vi "Lab Panel V5.31.vi"() -> ()   [LabVIEW 2017] (continued)
                            n1780 = local write "RUN LAB05-2"(w3330) -> ()
                            n1781 = local write "O/I  LAB05-2"(w3330) -> ()
                            n1782 = local write "run lab05-2"(w3330) -> ()
                            n1783 = local write "DISP LAB05-2"(w3333) -> ()
                          }
                          frame #1 {
                            n1784 = TDMS Close(11:w3334) -> (0:w3335:errorcluster)  [unwired: 1 in, 1 out]
                            n1785 = local write "data file error"(w3335) -> ()
                          }
                          frame #2 {
                            n1786 = stacked-sequence {
                              tunnel: "LAB05-2" -> [w3343 w3349]
                              tunnel: w3340 -> [_ w3348]
                              tunnel: w3339 -> [_ w3347]
                              tunnel: w3338 -> [_ w3346]
                              tunnel: w3337 -> [_ w3345]
                              tunnel: w3336 -> [_ w3344]
                              frame #0 {
                                n1787 = call "sub vi - defrag tdms v1.vi"("panel id"=w3343) -> ("error out"=w3342:errorcluster)  [unwired: 10 in]
                                n1788 = local write "data file error"(w3342) -> ()
                              }
                              frame #1 {
                                n1789 = Bundle("STATUS"=w3348, "OUT SERVER ADDRESS"=w3347, "FROM ACCOUNT"=w3346, "Mail Test File To:"=w3345, "Mail Test Fail"=w3344) -> (w3351:T29)  [unwired: 1 in]
                                n1790 = call "Save data file (pass-fail) v5.vi"("Input Cluster"=w3351, "panel id"=w3349) -> ("network file save error"=w3350:errorcluster)  [unwired: 8 in, 1 out]
                                n1791 = local write "data file error"(w3350) -> ()
                              }
                            }
                          }
                        }
                      }
                    }
                  }
                }
              }
            }
            n1792 = global write "Global display 2.vi" "Mail test file to:"(w2858) -> ()
            n1793 = local read "Network Directory"() -> (w2864:path)
            n1794 = global write "Global 1.vi" "Network Drive"(w2864) -> ()
          }
          frame #8 {
            # "disable functions"
            n1795 = stacked-sequence {
              tunnel: w3361 -> [w3375 _ w3432]
              tunnel: w3360 -> [w3370 _ w3431]
              tunnel: w3359 -> [w3369 _ w3430]
              tunnel: w3358 -> [w3367 _ w3429]
              tunnel: w3357 -> [w3368 _ w3428]
              tunnel: w3356 -> [_ w3392 w3427]
              tunnel: w3355 -> [_ w3393 w3426]
              tunnel: w3354 -> [_ w3394 w3425]
              tunnel: w3353 -> [_ w3395 w3424]
              tunnel: w3352 -> [_ w3396 w3423]
              frame #0 {
                n1796 = Select(t=2, s=w3367, f=0) -> (s? t:f=w3363:i32)
                n1797 = Select(t=2, s=w3369, f=0) -> (s? t:f=w3364:i32)
                n1798 = Select(t=2, s=w3368, f=0) -> (s? t:f=w3362:i32)
                n1799 = Select(t=2, s=w3375, f=0) -> (s? t:f=w3366:i32)
                n1800 = Select(t=2, s=w3370, f=0) -> (s? t:f=w3365:i32)
                n1801 = property on="SELECT LAB02-2" class="RadioBtnsControl (strict)"("DisabledEnum"=w3363) -> ()  [unwired: 2 in, 2 out]
                n1802 = property on="SELECT LAB02-1" class="RadioBtnsControl (strict)"("DisabledEnum"=w3364) -> ()  [unwired: 2 in, 2 out]
                n1803 = property on="SELECT LAB03-1" class="RadioBtnsControl (strict)"("DisabledEnum"=w3362) -> ()  [unwired: 2 in, 2 out]
                n1804 = property on="SELECT LAB01-1" class="RadioBtnsControl (strict)"("DisabledEnum"=w3366) -> ()  [unwired: 2 in, 2 out]
                n1805 = property on="SELECT LAB01-2" class="RadioBtnsControl (strict)"("DisabledEnum"=w3365) -> ()  [unwired: 2 in, 2 out]
                n1806 = Not(x=w3375) -> (.not. x?=w3376:bool)
                n1807 = property on="RESULT LAB01-1" class="Bool (strict)"("Visible"=w3376) -> ()  [unwired: 2 in, 2 out]
                n1808 = Not(x=w3370) -> (.not. x?=w3374:bool)
                n1809 = Not(x=w3369) -> (.not. x?=w3373:bool)
                n1810 = Not(x=w3367) -> (.not. x?=w3372:bool)
                n1811 = property on="RESULT LAB01-2" class="Bool (strict)"("Visible"=w3374) -> ()  [unwired: 2 in, 2 out]
                n1812 = Not(x=w3368) -> (.not. x?=w3371:bool)
                n1813 = property on="RESULT LAB02-1" class="Bool (strict)"("Visible"=w3373) -> ()  [unwired: 2 in, 2 out]
                n1814 = property on="RESULT LAB02-2" class="Bool (strict)"("Visible"=w3372) -> ()  [unwired: 2 in, 2 out]
                n1815 = property on="RESULT LAB03-1" class="Bool (strict)"("Visible"=w3371) -> ()  [unwired: 2 in, 2 out]
                n1816 = property on="SET LAB01-1" class="Clust (strict)"("DisabledEnum"=w3366) -> ()  [unwired: 2 in, 2 out]
                n1817 = property on="SET LAB01-2" class="Clust (strict)"("DisabledEnum"=w3365) -> ()  [unwired: 2 in, 2 out]
                n1818 = property on="SET LAB02-1" class="Clust (strict)"("DisabledEnum"=w3364) -> ()  [unwired: 2 in, 2 out]
                n1819 = property on="SET LAB02-2" class="Clust (strict)"("DisabledEnum"=w3363) -> ()  [unwired: 2 in, 2 out]
                n1820 = property on="SET LAB03-1" class="Clust (strict)"("DisabledEnum"=w3362) -> ()  [unwired: 2 in, 2 out]
                n1821 = property on="O/I  LAB01-1" class="Bool (strict)"("DisabledEnum"=w3366) -> ()  [unwired: 2 in, 2 out]
                n1822 = property on="O/I  LAB01-2" class="Bool (strict)"("DisabledEnum"=w3365) -> ()  [unwired: 2 in, 2 out]
                n1823 = property on="O/I  LAB02-1" class="Bool (strict)"("DisabledEnum"=w3364) -> ()  [unwired: 2 in, 2 out]
                n1824 = property on="O/I  LAB02-2" class="Bool (strict)"("DisabledEnum"=w3363) -> ()  [unwired: 2 in, 2 out]
                n1825 = property on="O/I  LAB03-1" class="Bool (strict)"("DisabledEnum"=w3362) -> ()  [unwired: 2 in, 2 out]
              }
              frame #1 {
                n1826 = Select(t=2, s=w3396, f=0) -> (s? t:f=w3387:i32)
                n1827 = Select(t=2, s=w3395, f=0) -> (s? t:f=w3388:i32)
                n1828 = Select(t=2, s=w3392, f=0) -> (s? t:f=w3391:i32)
                n1829 = Select(t=2, s=w3393, f=0) -> (s? t:f=w3390:i32)
                n1830 = Select(t=2, s=w3394, f=0) -> (s? t:f=w3389:i32)
                n1831 = property on="SELECT LAB05-2" class="RadioBtnsControl (strict)"("DisabledEnum"=w3387) -> ()  [unwired: 2 in, 2 out]
                n1832 = property on="SELECT LAB05-1" class="RadioBtnsControl (strict)"("DisabledEnum"=w3388) -> ()  [unwired: 2 in, 2 out]
                n1833 = property on="SELECT LAB03-2" class="RadioBtnsControl (strict)"("DisabledEnum"=w3391) -> ()  [unwired: 2 in, 2 out]
                n1834 = property on="SELECT LAB04-1" class="RadioBtnsControl (strict)"("DisabledEnum"=w3390) -> ()  [unwired: 2 in, 2 out]
                n1835 = property on="SELECT LAB04-2" class="RadioBtnsControl (strict)"("DisabledEnum"=w3389) -> ()  [unwired: 2 in, 2 out]
                n1836 = property on="SET LAB05-2" class="Clust (strict)"("DisabledEnum"=w3387) -> ()  [unwired: 2 in, 2 out]
                n1837 = property on="SET LAB05-1" class="Clust (strict)"("DisabledEnum"=w3388) -> ()  [unwired: 2 in, 2 out]
                n1838 = property on="SET LAB03-2" class="Clust (strict)"("DisabledEnum"=w3391) -> ()  [unwired: 2 in, 2 out]
                n1839 = property on="SET LAB04-1" class="Clust (strict)"("DisabledEnum"=w3390) -> ()  [unwired: 2 in, 2 out]
                n1840 = property on="SET LAB04-2" class="Clust (strict)"("DisabledEnum"=w3389) -> ()  [unwired: 2 in, 2 out]
                n1841 = property on="O/I  LAB05-2" class="Bool (strict)"("DisabledEnum"=w3387) -> ()  [unwired: 2 in, 2 out]
                n1842 = property on="O/I  LAB05-1" class="Bool (strict)"("DisabledEnum"=w3388) -> ()  [unwired: 2 in, 2 out]
                n1843 = property on="O/I  LAB04-1" class="Bool (strict)"("DisabledEnum"=w3390) -> ()  [unwired: 2 in, 2 out]
                n1844 = property on="O/I  LAB04-2" class="Bool (strict)"("DisabledEnum"=w3389) -> ()  [unwired: 2 in, 2 out]
                n1845 = property on="O/I  LAB03-2" class="Bool (strict)"("DisabledEnum"=w3391) -> ()  [unwired: 2 in, 2 out]
                n1846 = Not(x=w3396) -> (.not. x?=w3397:bool)
                n1847 = Not(x=w3395) -> (.not. x?=w3398:bool)
                n1848 = Not(x=w3394) -> (.not. x?=w3399:bool)
                n1849 = property on="RESULT LAB05-2" class="Bool (strict)"("Visible"=w3397) -> ()  [unwired: 2 in, 2 out]
                n1850 = property on="RESULT LAB05-1" class="Bool (strict)"("Visible"=w3398) -> ()  [unwired: 2 in, 2 out]
                n1851 = Not(x=w3393) -> (.not. x?=w3400:bool)
                n1852 = property on="RESULT LAB04-2" class="Bool (strict)"("Visible"=w3399) -> ()  [unwired: 2 in, 2 out]
                n1853 = Not(x=w3392) -> (.not. x?=w3401:bool)
                n1854 = property on="RESULT LAB04-1" class="Bool (strict)"("Visible"=w3400) -> ()  [unwired: 2 in, 2 out]
                n1855 = property on="RESULT LAB03-2" class="Bool (strict)"("Visible"=w3401) -> ()  [unwired: 2 in, 2 out]
              }
              frame #2 {
                # "disable calibrate if any test running"
                n1856 = Or(x=w3424, y=w3423) -> (x .or. y?=w3417:bool)
                n1857 = Or(x=w3426, y=w3425) -> (x .or. y?=w3419:bool)
                n1858 = Or(x=w3430, y=w3429) -> (x .or. y?=w3421:bool)
                n1859 = Or(x=w3428, y=w3427) -> (x .or. y?=w3420:bool)
                n1860 = Or(x=w3432, y=w3431) -> (x .or. y?=w3422:bool)
                n1861 = Or(x=w3420, y=w3419) -> (x .or. y?=w3418:bool)
                n1862 = Or(x=w3422, y=w3421) -> (x .or. y?=w3416:bool)
                n1863 = Or(x=w3418, y=w3417) -> (x .or. y?=w3415:bool)
                n1864 = Or(x=w3416, y=w3415) -> (x .or. y?=w3412:bool)
                "Any Test Running" <- w3412
                n1865 = case shown="False" w3412 {
                  tunnel: [0 2] -> w3414
                  frame False {
                  }
                  frame True {
                  }
                }
                n1866 = property on="JIG TEST" class="Clust (strict)"("DisabledEnum"=w3414) -> ()  [unwired: 2 in, 2 out]
                n1867 = property on="Network Directory" class="Path"("DisabledEnum"=w3414) -> ()  [unwired: 2 in, 2 out]
                n1868 = property on="MAIL SETTINGS" class="Clust (strict)"("DisabledEnum"=w3414) -> ()  [unwired: 2 in, 2 out]
                n1869 = property on="SET (cal)" class="Bool (strict)"("DisabledEnum"=w3414) -> ()  [unwired: 2 in, 2 out]
                n1870 = property on="ADMIN" class="Bool (strict)"("DisabledEnum"=0) -> ()  [unwired: 2 in, 2 out]
              }
            }
          }
          frame #9 {
            # "Note : JIG LAB0X-N   are written to digital I/O in frame 11"
            # "Drive jigs"
            n1871 = stacked-sequence {
              frame #0 {
                # "jig on"
                n1872 = local read "jig cycle"() -> (w3440:dbl)
                n1873 = property on="JIG TEST" class="Clust (strict)"() -> ("DisabledEnum"=w3437:T17)  [unwired: 2 in, 2 out]
                n1874 = Equal?(x=w3437, y=2) -> (x = y?=w3436:bool)
                n1875 = Equal?(x=w3440, y=0) -> (x = y?=w3438:bool)
                n1876 = And(x=w3438, y=w3436) -> (x .and. y?=w3435:bool)
                n1877 = case shown="True" w3435 {
                  frame False {
                  }
                  frame True {
                    n1878 = local read "run lab01-2"() -> (w3450:bool)
                    n1879 = local read "run lab01-1"() -> (w3451:bool)
                    n1880 = local read "run lab02-1"() -> (w3449:bool)
                    n1881 = local read "run lab02-2"() -> (w3448:bool)
                    n1882 = local read "run lab03-1"() -> (w3447:bool)
                    n1883 = local read "run lab03-2"() -> (w3446:bool)
                    n1884 = local read "run lab04-1"() -> (w3445:bool)
                    n1885 = local read "run lab04-2"() -> (w3444:bool)
                    n1886 = local read "run lab05-1"() -> (w3443:bool)
                    n1887 = local read "run lab05-2"() -> (w3442:bool)
                    n1888 = local write "JIG LAB01-2"(w3450) -> ()
                    n1889 = local write "JIG LAB03-2"(w3446) -> ()
                    n1890 = local write "JIG LAB01-1"(w3451) -> ()
                    n1891 = local write "JIG LAB02-1"(w3449) -> ()
                    n1892 = local write "JIG LAB02-2"(w3448) -> ()
                    n1893 = local write "JIG LAB03-1"(w3447) -> ()
                    n1894 = local write "JIG LAB04-1"(w3445) -> ()
                    n1895 = local write "JIG LAB04-2"(w3444) -> ()
                    n1896 = local write "JIG LAB05-1"(w3443) -> ()
                    n1897 = local write "JIG LAB05-2"(w3442) -> ()
                  }
                }
              }
              frame #1 {
                # "jig off"
                n1898 = local read "jig cycle"() -> (w3458:dbl)
                n1899 = local read "on loops"() -> (w3457:dbl)
                n1900 = property on="JIG TEST" class="Clust (strict)"() -> ("DisabledEnum"=w3456:T17)  [unwired: 2 in, 2 out]
                n1901 = Equal?(x=w3456, y=2) -> (x = y?=w3454:bool)
                n1902 = Equal?(x=w3458, y=w3457) -> (x = y?=w3453:bool)
                n1903 = And(x=w3453, y=w3454) -> (x .and. y?=w3452:bool)
                n1904 = case shown="True" w3452 {
                  frame False {
                  }
                  frame True {
                    w3509 = FALSE
                    w3510 = TRUE
                    w3508 = 2
                    n1905 = local read "SELECT LAB05-2"() -> (w3499:T3)
                    n1906 = local read "SELECT LAB04-2"() -> (w3501:T3)
                    n1907 = local read "SELECT LAB04-1"() -> (w3502:T3)
                    n1908 = local read "SELECT LAB05-1"() -> (w3500:T3)
                    n1909 = local read "SELECT LAB03-2"() -> (w3503:T3)
                    n1910 = local read "SELECT LAB02-1"() -> (w3506:T3)
                    n1911 = local read "SELECT LAB03-1"() -> (w3504:T3)
                    n1912 = local read "SELECT LAB02-2"() -> (w3505:T3)
                    n1913 = local read "SELECT LAB01-2"() -> (w3507:T3)
                    n1914 = local read "run lab05-1"() -> (w3469:bool)
                    n1915 = local read "run lab05-2"() -> (w3468:bool)
                    n1916 = local read "run lab04-2"() -> (w3470:bool)
                    n1917 = local read "SELECT LAB01-1"() -> (w3511:T3)
                    n1918 = local read "run lab04-1"() -> (w3471:bool)
                    n1919 = local read "run lab01-1"() -> (w3487:bool)
                    n1920 = local read "run lab01-2"() -> (w3476:bool)
                    n1921 = local read "run lab03-2"() -> (w3472:bool)
                    n1922 = local read "run lab03-1"() -> (w3473:bool)
                    n1923 = local read "run lab02-1"() -> (w3475:bool)
                    n1924 = local read "run lab02-2"() -> (w3474:bool)
                    n1925 = Equal?(x=w3508, y=w3504) -> (x = y?=w3482:bool)
                    n1926 = Equal?(x=w3508, y=w3503) -> (x = y?=w3481:bool)
                    n1927 = Equal?(x=w3508, y=w3502) -> (x = y?=w3480:bool)
                    n1928 = Equal?(x=w3508, y=w3501) -> (x = y?=w3479:bool)
                    n1929 = Equal?(x=w3508, y=w3500) -> (x = y?=w3478:bool)
                    n1930 = Equal?(x=w3508, y=w3499) -> (x = y?=w3477:bool)
                    n1931 = Equal?(x=w3508, y=w3511) -> (x = y?=w3488:bool)
                    n1932 = Equal?(x=w3508, y=w3506) -> (x = y?=w3484:bool)
                    n1933 = Equal?(x=w3508, y=w3505) -> (x = y?=w3483:bool)
                    n1934 = Equal?(x=w3508, y=w3507) -> (x = y?=w3485:bool)
                    n1935 = And(x=w3479, y=w3470) -> (x .and. y?=w3461:bool)
                    n1936 = And(x=w3482, y=w3473) -> (x .and. y?=w3464:bool)
                    n1937 = And(x=w3480, y=w3471) -> (x .and. y?=w3462:bool)
                    n1938 = And(x=w3477, y=w3468) -> (x .and. y?=w3459:bool)
                    n1939 = And(x=w3483, y=w3474) -> (x .and. y?=w3465:bool)
                    n1940 = And(x=w3481, y=w3472) -> (x .and. y?=w3463:bool)
                    n1941 = And(x=w3478, y=w3469) -> (x .and. y?=w3460:bool)
                    n1942 = And(x=w3485, y=w3476) -> (x .and. y?=w3467:bool)
                    n1943 = And(x=w3488, y=w3487) -> (x .and. y?=w3486:bool)
                    n1944 = And(x=w3484, y=w3475) -> (x .and. y?=w3466:bool)
                    n1945 = Select(t=w3510, s=w3486, f=w3509) -> (s? t:f=w3489:bool)
                    n1946 = Select(t=w3510, s=w3467, f=w3509) -> (s? t:f=w3490:bool)
                    n1947 = Select(t=w3510, s=w3466, f=w3509) -> (s? t:f=w3491:bool)
                    n1948 = Select(t=w3510, s=w3465, f=w3509) -> (s? t:f=w3492:bool)
                    n1949 = Select(t=w3510, s=w3464, f=w3509) -> (s? t:f=w3493:bool)
                    n1950 = Select(t=w3510, s=w3463, f=w3509) -> (s? t:f=w3494:bool)
                    n1951 = Select(t=w3510, s=w3462, f=w3509) -> (s? t:f=w3495:bool)
                    n1952 = Select(t=w3510, s=w3461, f=w3509) -> (s? t:f=w3496:bool)
                    n1953 = Select(t=w3510, s=w3460, f=w3509) -> (s? t:f=w3497:bool)
                    n1954 = Select(t=w3510, s=w3459, f=w3509) -> (s? t:f=w3498:bool)
                    n1955 = local write "JIG LAB03-2"(w3494) -> ()
                    n1956 = local write "JIG LAB02-1"(w3491) -> ()
                    n1957 = local write "JIG LAB02-2"(w3492) -> ()
                    n1958 = local write "JIG LAB01-2"(w3490) -> ()
                    n1959 = local write "JIG LAB03-1"(w3493) -> ()
                    n1960 = local write "JIG LAB01-1"(w3489) -> ()
                    n1961 = local write "JIG LAB05-2"(w3498) -> ()
                    n1962 = local write "JIG LAB04-1"(w3495) -> ()
                    n1963 = local write "JIG LAB05-1"(w3497) -> ()
                    n1964 = local write "JIG LAB04-2"(w3496) -> ()
                  }
                }
              }
            }
          }
          frame #10 {
            # "Note : JIG LAB0X-N   are written to digital I/O in frame 11"
            # "enable  jig test output if no test busy"
            n1965 = property on="JIG TEST" class="Clust (strict)"() -> ("DisabledEnum"=w3514:T17)  [unwired: 2 in, 2 out]
            n1966 = Equal?(x=w3514, y=0) -> (x = y?=w3512:bool)
            n1967 = case shown="True" w3512 {
              frame False {
              }
              frame True {
                n1968 = local read "JIG TEST"() -> (w3525:T11)
                n1969 = Unbundle(w3525) -> ("LAB01-1"=w3524:bool, "LAB01-2"=w3523:bool, "LAB02-1"=w3522:bool, "LAB02-2"=w3521:bool, "LAB03-1"=w3520:bool, "LAB03-2"=w3519:bool, "LAB04-1"=w3518:bool, "LAB04-2"=w3517:bool, "LAB05-1"=w3516:bool, "LAB05-2"=w3515:bool)
                n1970 = local write "JIG LAB05-1"(w3516) -> ()
                n1971 = local write "JIG LAB05-2"(w3515) -> ()
                n1972 = local write "JIG LAB04-1"(w3518) -> ()
                n1973 = local write "JIG LAB04-2"(w3517) -> ()
                n1974 = local write "JIG LAB03-2"(w3519) -> ()
                n1975 = local write "JIG LAB01-1"(w3524) -> ()
                n1976 = local write "JIG LAB02-1"(w3522) -> ()
                n1977 = local write "JIG LAB03-1"(w3520) -> ()
                n1978 = local write "JIG LAB01-2"(w3523) -> ()
                n1979 = local write "JIG LAB02-2"(w3521) -> ()
              }
            }
          }
          frame #11 {
            w3526 = FALSE
            # "Drive digital output and reset USB and temperature network if required."
            n1980 = global read "Global display 3.vi" "cycle O/F"() -> (w3535:bool)
            n1981 = case shown="False" w3535 {
              tunnel: [w3667 FALSE] -> w3534
              frame False {
                n1982 = local read "Analog error"() -> (w3669:bool)
                n1983 = local read "Reset Measuring"() -> (w3668:bool)
                n1984 = Or(x=w3668, y=w3669) -> (x .or. y?=w3667:bool)
              }
              frame True {
              }
            }
            n1985 = local read "O/I  LAB01-1"() -> (w3554:bool)
            n1986 = local read "JIG LAB01-1"() -> (w3553:bool)
            n1987 = local read "O/I  LAB01-2"() -> (w3552:bool)
            n1988 = local read "JIG LAB01-2"() -> (w3551:bool)
            n1989 = local read "O/I  LAB02-1"() -> (w3550:bool)
            n1990 = local read "JIG LAB02-1"() -> (w3549:bool)
            n1991 = local read "O/I  LAB02-2"() -> (w3548:bool)
            n1992 = local read "JIG LAB02-2"() -> (w3547:bool)
            n1993 = local read "O/I  LAB03-1"() -> (w3546:bool)
            n1994 = local read "JIG LAB03-1"() -> (w3545:bool)
            n1995 = local read "O/I  LAB03-2"() -> (w3544:bool)
            n1996 = local read "JIG LAB03-2"() -> (w3543:bool)
            n1997 = local read "O/I  LAB04-1"() -> (w3542:bool)
            n1998 = local read "JIG LAB04-1"() -> (w3541:bool)
            n1999 = local read "O/I  LAB04-2"() -> (w3532:bool)
            n2000 = local read "JIG LAB04-2"() -> (w3531:bool)
            n2001 = local read "O/I  LAB05-1"() -> (w3530:bool)
            n2002 = local read "JIG LAB05-1"() -> (w3529:bool)
            n2003 = local read "O/I  LAB05-2"() -> (w3528:bool)
            n2004 = local read "JIG LAB05-2"() -> (w3527:bool)
            n2005 = Build Array(w3547, w3546, w3545, w3544, w3543, w3542, w3541) -> (w3539:bool[])
            "USB OUT 1" <- w3539
            n2006 = Build Array(w3554, w3553, w3552, w3551, w3550, w3549, w3548) -> (w3540:bool[])
            "USB OUT 0" <- w3540
            n2007 = Build Array(w3532, w3531, w3530, w3529, w3528, w3527, w3526, w3526) -> (w3538:bool[])
            "USB OUT 2" <- w3538
            n2008 = Not(x=w3535) -> (.not. x?=w3536:bool)
            n2009 = local read "Simulate"() -> (w3537:bool)
            n2010 = And(x=w3536, y=w3534) -> (x .and. y?=w3533:bool)
            n2011 = stacked-sequence {
              tunnel: w3540 -> [w3558 w3564]
              tunnel: w3539 -> [w3557 w3563]
              tunnel: w3538 -> [w3556 w3562]
              tunnel: w3537 -> [w3555 w3565]
              tunnel: w3533 -> [_ w3566]
              frame #0 {
                # "drive outputs for normal use"
                n2012 = case shown="False" w3555 {
                  tunnel: w3558 -> [w3561 _]
                  tunnel: w3557 -> [w3560 _]
                  tunnel: w3556 -> [w3559 _]
                  frame False {
                    n2013 = call "sub vi - Drive Relays All v6.vi"("Array #2"=w3559, "Array #1"=w3560, "Array #0"=w3561) -> ()  [unwired: 8 in, 1 out]
                  }
                  frame True {
                  }
                }
              }
              frame #1 {
                # "USB  reset routine"
                n2014 = case shown="True" w3566 {
                  tunnel: w3565 -> [_ w3570]
                  tunnel: w3564 -> [_ w3569]
                  tunnel: w3563 -> [_ w3568]
                  tunnel: w3562 -> [_ w3567]
                  frame False {
                  }
                  frame True {
                    n2015 = stacked-sequence {
                      seq-local: [w3572 _ _ _ _] -> [_ w3578 _ _ _]
                      tunnel: w3570 -> [_ w3582 _ _ _]
                      tunnel: w3569 -> [_ w3581 _ _ _]
                      tunnel: w3568 -> [_ w3580 _ _ _]
                      tunnel: w3567 -> [_ w3579 _ _ _]
                      frame #0 {
                        n2016 = case shown="False" "Auto Reset" {
                          tunnel: [w3575 FALSE] -> w3573
                          frame False {
                            n2017 = Two Button Dialog(message="System reset") -> (T button?=w3575:bool)  [unwired: 2 in]
                          }
                          frame True {
                          }
                        }
                        n2018 = disable-structure shown="Disabled" {
                          frame Disabled {
                            n2019 = local write "Tab Control 2"(5) -> ()
                          }
                          frame Enabled {
                          }
                        }
                        n2020 = Or(x="Auto Reset", y=w3573) -> (x .or. y?=w3572:bool)
                      }
                      frame #1 {
                        n2021 = case shown="True" w3578 {
                          tunnel: w3582 -> [_ w3588]
                          tunnel: w3581 -> [_ w3587]
                          tunnel: w3580 -> [_ w3586]
                          tunnel: w3579 -> [_ w3585]
                          frame False {
                          }
                          frame True {
                            n2022 = stacked-sequence {
                              tunnel: w3588 -> [_ w3606 _]
                              tunnel: bool[] [] -> [w3591 w3605 w3624]
                              tunnel: w3587 -> [_ _ w3623]
                              tunnel: w3586 -> [w3590 _ w3622]
                              tunnel: w3585 -> [w3589 _ w3621]
                              tunnel: 5000 -> [w3592 _ w3620]
                              frame #0 {
                                # "switch off test stations for system reset"
                                n2023 = stacked-sequence {
                                tunnel: w3592 -> [w3596 w3600 w3602]
                                tunnel: w3591 -> [w3595 w3599 w3603]
                                tunnel: w3590 -> [w3594 _ _]
                                tunnel: w3589 -> [w3593 w3598 _]
                                frame #0 {
                                # "drive 1st 7 inputs"
                                n2024 = call "sub vi - Drive Relays All v6.vi"("Array #2"=w3593, "Array #1"=w3594, "Array #0"=w3595) -> ()  [unwired: 8 in, 1 out]
                                n2025 = call "Message Display V1.vi"("Message"="Delay off LAB 01-1 to 02-1", "Delay mS"=w3596) -> ()  [unwired: 10 in]
                                }
                                frame #1 {
                                # "drive 2nd 7 inputs"
                                n2026 = call "sub vi - Drive Relays All v6.vi"("Array #2"=w3598, "Array #1"=w3599, "Array #0"=w3599) -> ()  [unwired: 8 in, 1 out]
                                n2027 = call "Message Display V1.vi"("Message"="Delay off LAB 02-2 to 04-1", "Delay mS"=w3600) -> ()  [unwired: 10 in]
                                }
                                frame #2 {
                                # "drive 3rd 7 inputs"
                                n2028 = call "sub vi - Drive Relays All v6.vi"("Array #2"=w3603, "Array #1"=w3603, "Array #0"=w3603) -> ()  [unwired: 8 in, 1 out]
                                n2029 = call "Message Display V1.vi"("Message"="Delay off LAB 04-2 to 05-2", "Delay mS"=w3602) -> ()  [unwired: 10 in]
                                }
                                }
                              }
                              frame #1 {
                                # "reset all usb modules"
                                n2030 = stacked-sequence {
                                tunnel: w3606 -> [_ w3611]
                                tunnel: w3605 -> [w3609 _]
                                frame #0 {
                                n2031 = local write "AI Task"(FALSE) -> ()
                                n2032 = call "sub vi - Drive Relays All v6.vi"("Array #2"=bool[] [FALSE, FALSE, FALSE, FALSE, FALSE, FALSE, TRUE, FALSE], "Array #1"=w3609, "Array #0"=w3609) -> ()  [unwired: 8 in, 1 out]
                                }
                                frame #1 {
                                n2033 = call "Reset Meas v 5.vi"("simulate"=w3611) -> ("Reset Error"=w3610:bool)  [unwired: 10 in]
                                n2034 = case shown="False" w3610 {
                                frame False {
                                n2035 = local read "RATE (Hz)"() -> (w3615:dbl)
                                n2036 = local read "SAMPLES"() -> (w3614:dbl)
                                n2037 = call "sub vi - AI USB4704 (3)  Create Task v4.vi"("Rate Hz"=w3615, "Samples"=w3614) -> ("TASK USB 0"=w3618:i32, "TASK USB 1"=w3617:i32, "TASK USB 2"=w3616:i32, "AI Task Er"=w3612:bool)  [unwired: 9 in, 1 out]
                                n2038 = local write "AI Task"(TRUE) -> ()
                                n2039 = local write "Reset Error"(w3612) -> ()
                                n2040 = local write "AI Task2"(w3616) -> ()
                                n2041 = local write "AI Task1"(w3617) -> ()
                                n2042 = local write "AI Task0"(w3618) -> ()
                                }
                                frame True {
                                "Reset Error" <- TRUE
                                }
                                }
                                }
                                }
                              }
                              frame #2 {
                                # "switch test stations back on after reset"
                                n2043 = stacked-sequence {
                                tunnel: w3624 -> [w3628 w3631 _]
                                tunnel: w3623 -> [w3627 w3633 w3638]
                                tunnel: w3620 -> [w3626 w3629 w3635]
                                tunnel: w3622 -> [_ w3632 w3637]
                                tunnel: w3621 -> [_ _ w3634]
                                frame #0 {
                                # "drive 1st 7 inputs"
                                n2044 = call "sub vi - Drive Relays All v6.vi"("Array #2"=w3628, "Array #1"=w3628, "Array #0"=w3627) -> ()  [unwired: 8 in, 1 out]
                                n2045 = call "Message Display V1.vi"("Message"="Delay on LAB 01-1 to 02-1", "Delay mS"=w3626) -> ()  [unwired: 10 in]
                                }
                                frame #1 {
                                # "drive 1st & 2nd outputs"
                                n2046 = call "sub vi - Drive Relays All v6.vi"("Array #2"=w3631, "Array #1"=w3632, "Array #0"=w3633) -> ()  [unwired: 8 in, 1 out]
                                n2047 = call "Message Display V1.vi"("Message"="Delay on LAB 02-2 to 04-1", "Delay mS"=w3629) -> ()  [unwired: 10 in]
                                }
                                frame #2 {
                                n2048 = call "sub vi - Drive Relays All v6.vi"("Array #2"=w3634, "Array #1"=w3637, "Array #0"=w3638) -> ()  [unwired: 8 in, 1 out]
                                n2049 = call "Message Display V1.vi"("Message"="Delay on LAB 04-2 to 05-2", "Delay mS"=w3635) -> ()  [unwired: 10 in]
                                }
                                }
                              }
                            }
                          }
                        }
                      }
                      frame #2 {
                        w3639 = 0
                        w3640 = FALSE
                        # "set all back to zero"
                        n2050 = local read "Total USB resets"() -> (w3642:dbl)
                        n2051 = local read "Resets Done"() -> (w3644:dbl)
                        n2052 = local write "Reset Measuring"(w3640) -> ()
                        n2053 = local write "Analog error"(w3640) -> ()
                        n2054 = local write "Er USB#2"(w3639) -> ()
                        n2055 = local write "Er USB#0"(w3639) -> ()
                        n2056 = local write "Er USB#1"(w3639) -> ()
                        n2057 = local write "Error USB #0"(w3640) -> ()
                        n2058 = local write "Error USB #1"(w3640) -> ()
                        n2059 = local write "Error USB #2"(w3640) -> ()
                        n2060 = Increment(x=w3642) -> (x+1=w3641:dbl)
                        n2061 = Increment(x=w3644) -> (x+1=→"Resets Done":dbl)
                        n2062 = local write "Total USB resets"(w3641) -> ()
                      }
                      frame #3 {
                        # "save reset value"
                        n2063 = String To Path(string="c:\\crabtree\\Set Up\\") -> (path=w3654:path)
                        n2064 = Build Path(base path=w3654, name or relative path="USB resets.bin") -> (appended path=w3647:path)
                        n2065 = Create Folder(path (use dialog)=w3654) -> (error out=w3646:errorcluster)  [unwired: 2 in, 2 out]
                        n2066 = local read "Total USB resets"() -> (w3645:dbl)
                        n2067 = call <vilib>:"Clear Errors.vi"("error in (no error)"=w3646) -> ()  [unwired: 5 in, 2 out]
                        n2068 = Open/Create/Replace File(file path (use dialog)=w3647, operation (0:open)=T18."replace or create") -> (refnum out=w3652:refnum<file>, error out=w3651:errorcluster)  [unwired: 4 in, 1 out]
                        n2069 = Write to Binary File(file (use dialog)=w3652, data=w3645, error in=w3651) -> (refnum out=w3650:refnum<file>, error out=w3649:errorcluster)  [unwired: 3 in, 1 out]
                        n2070 = Close File(refnum=w3650, error in=w3649) -> (error out=w3648:errorcluster)  [unwired: 1 out]
                        n2071 = local write "data file error"(w3648) -> ()
                      }
                      frame #4 {
                        # "mail reset value"
                        n2072 = local read "MAIL SETTINGS"() -> (w3660:T8)
                        n2073 = local read "Total USB resets"() -> (w3664:dbl)
                        n2074 = Unbundle(w3660) -> ("OUT SERVER ADDRESS"=w3666:string, "FROM ACCOUNT"=w3665:string)  [unwired: 5 out]
                        n2075 = Number To Decimal String(number=w3664) -> (decimal integer string=w3662:string)  [unwired: 1 in]
                        n2076 = Concatenate Strings("Total USB resets: ", w3662) -> (w3661:string)
                        n2077 = call "sub vi - send mail v5.vi"("TO:"="francois@ffg.net", "subject"=w3661, "from"=w3665, "out going server"=w3666) -> ("error out"=w3659:errorcluster)  [unwired: 11 in]
                        n2078 = Bundle(cluster=w3660, "mail error"=w3659) -> (w3658:T8)  [unwired: 6 in]
                        n2079 = local write "MAIL SETTINGS"(w3658) -> ()
                      }
                    }
                  }
                }
              }
            }
          }
          frame #12 {
            # "if all test panels are off stop analog read"
            n2080 = local read "O/I  LAB03-1"() -> (w3692:bool)
            n2081 = local read "O/I  LAB03-2"() -> (w3691:bool)
            n2082 = local read "O/I  LAB04-1"() -> (w3690:bool)
            n2083 = local read "O/I  LAB04-2"() -> (w3689:bool)
            n2084 = local read "O/I  LAB05-1"() -> (w3688:bool)
            n2085 = local read "O/I  LAB05-2"() -> (w3687:bool)
            n2086 = local read "O/I  LAB02-2"() -> (w3693:bool)
            n2087 = local read "O/I  LAB02-1"() -> (w3694:bool)
            n2088 = local read "O/I  LAB01-2"() -> (w3695:bool)
            n2089 = local read "O/I  LAB01-1"() -> (w3696:bool)
            n2090 = Or(x=w3688, y=w3687) -> (x .or. y?=w3685:bool)
            n2091 = Or(x=w3690, y=w3689) -> (x .or. y?=w3686:bool)
            n2092 = Or(x=w3694, y=w3693) -> (x .or. y?=w3684:bool)
            n2093 = Or(x=w3692, y=w3691) -> (x .or. y?=w3682:bool)
            n2094 = Or(x=w3696, y=w3695) -> (x .or. y?=w3683:bool)
            n2095 = Or(x=w3686, y=w3685) -> (x .or. y?=w3679:bool)
            n2096 = Or(x=w3683, y=w3684) -> (x .or. y?=w3681:bool)
            n2097 = Or(x=w3681, y=w3682) -> (x .or. y?=w3680:bool)
            n2098 = Or(x=w3680, y=w3679) -> (x .or. y?=w3677:bool)
            n2099 = local read "Any Test Running"() -> (w3678:bool)
            n2100 = local read "AI Task"() -> (w3673:bool)
            n2101 = Or(x=w3677, y=w3678) -> (x .or. y?=w3672:bool)
            n2102 = Not(x=w3672) -> (.not. x?=w3676:bool)
            n2103 = And(x=w3676, y=w3673) -> (x .and. y?=w3675:bool)
            n2104 = Not(x=w3673) -> (.not. x?=w3674:bool)
            n2105 = And(x=w3672, y=w3674) -> (x .and. y?=w3671:bool)
            n2106 = case shown="True" w3675 {
              frame False {
              }
              frame True {
                # "close task if no test"
                n2107 = local write "AI Task"(FALSE) -> ()
                n2108 = call "sub vi - AI USB4704 (3)  Close Task v2.vi"() -> ()  [unwired: 16 in]
              }
            }
            n2109 = case shown="True" w3671 {
              frame False {
              }
              frame True {
                # "create task for test"
                n2110 = local read "SAMPLES"() -> (w3698:dbl)
                n2111 = local read "RATE (Hz)"() -> (w3697:dbl)
                n2112 = call "sub vi - AI USB4704 (3)  Create Task v4.vi"("Rate Hz"=w3697, "Samples"=w3698) -> ("TASK USB 0"=w3699:i32, "TASK USB 1"=w3700:i32, "TASK USB 2"=w3701:i32)  [unwired: 9 in, 2 out]
                n2113 = local write "AI Task0"(w3699) -> ()
                n2114 = local write "AI Task1"(w3700) -> ()
                n2115 = local write "AI Task2"(w3701) -> ()
                n2116 = local write "AI Task"(TRUE) -> ()
              }
            }
          }
          frame #13 {
            # "get all analog values from USB devices"
            n2117 = local read "on loops"() -> (w3711:dbl)
            n2118 = local read "jig cycle"() -> (w3708:dbl)
            n2119 = Add(x=w3711, y=3) -> (x+y=w3709:dbl)
            n2120 = Equal?(x=w3708, y=3) -> (x = y?=w3706:bool)
            n2121 = Equal?(x=w3708, y=w3709) -> (x = y?=w3707:bool)
            n2122 = Or(x=w3706, y=w3707) -> (x .or. y?=w3705:bool)
            n2123 = global write "Global display 3.vi" "cycle O/F"(w3706) -> ()
            n2124 = case shown="True" w3705 {
              tunnel: w3706 -> [_ w3717]
              tunnel: w3704 -> [_ w3714]
              frame False {
              }
              frame True {
                n2125 = local read "Simulate"() -> (w3720:bool)
                n2126 = case shown="False" w3720 {
                  tunnel: [w3736 dynamicdata[] [] ("array GRAPH")] -> w3726
                  tunnel: [w3735 w3761] -> w3725
                  tunnel: [w3734 w3761] -> w3724
                  tunnel: [w3733 w3761] -> w3723
                  tunnel: [w3732 w3761] -> w3722
                  tunnel: [w3731 w3761] -> w3721
                  tunnel: w3717 -> [_ w3765]
                  tunnel: [w3730 "Ambient Volts"] -> w3716
                  tunnel: [w3729 bool[] []] -> w3715
                  tunnel: w3714 -> [w3728 _]
                  tunnel: [w3727 0.3 ("Analog loop time")] -> w3713
                  frame False {
                    # "analog in"
                    n2127 = case shown="True" w3728 {
                      tunnel: [dynamicdata[] [] ("array GRAPH") w3755] -> w3736
                      tunnel: [w3738 w3754] -> w3735
                      tunnel: [w3738 w3753] -> w3734
                      tunnel: [w3738 w3752] -> w3733
                      tunnel: [w3738 w3751] -> w3732
                      tunnel: [w3738 w3750] -> w3731
                      tunnel: [3 w3749] -> w3730
                      tunnel: [bool[] [] w3748] -> w3729
                      tunnel: [0.0 w3744] -> w3727
                      frame False {
                        w3739 = 0.0
                        # "no test"
                        n2128 = Bundle(w3739, w3739, w3739, w3739, w3739, w3739) -> (w3738:cluster{dbl, dbl, dbl, dbl, dbl, dbl})  [unwired: 1 in]
                      }
                      frame True {
                        # "test on"
                        n2129 = local read "AI data 0"() -> (w3747:waveform(dbl)[])
                        n2130 = local read "AI data 1"() -> (w3746:waveform(dbl)[])
                        n2131 = local read "AI data 2"() -> (w3743:waveform(dbl)[])
                        n2132 = local read "AI Error"() -> (w3745:errorcluster[])
                        n2133 = call "sub vi - Read Analog All v9.5.vi"("data 0"=w3747, "data 1"=w3746, "data 2"=w3743, "AI Error"=w3745) -> ("array GRAPH"=w3755:dynamicdata[], "LAB01"=w3754:T30, "LAB02"=w3753:T31, "LAB03"=w3752:T32, "LAB04"=w3751:T33, "deg C"=w3749:dbl, "USB Error"=w3748:bool[], "LAB05"=w3750:T34)  [unwired: 4 in]
                        n2134 = local read "AI loop time"() -> (w3744:dbl)
                      }
                    }
                  }
                  frame True {
                    # "simulate"
                    n2135 = local read "ON amps"() -> (w3759:dbl)
                    n2136 = local read "OFF amps"() -> (w3760:dbl)
                    n2137 = local read "VOLTS"() -> (w3763:dbl)
                    n2138 = local read "PF"() -> (w3762:dbl)
                    n2139 = Select(t=w3759, s=w3765, f=w3760) -> (s? t:f=w3764:dbl)
                    n2140 = Bundle("OFF amps"=w3764, "VOLTS"=w3763, "PF"=w3762, "OFF amps"=w3764, "VOLTS"=w3763, "PF"=w3762) -> (w3761:T35)  [unwired: 1 in]
                  }
                }
                n2141 = local read "Simulate"() -> (w3719:bool)
                n2142 = stacked-sequence {
                  seq-local: [w3769 _ _ _ _ _ _ _] -> [_ _ _ _ _ _ _ _]
                  seq-local: [w3768 _ _ _ _ _ _ _] -> [_ _ _ _ _ _ _ _]
                  seq-local: [w3767 _ _ _ _ _ _ _] -> [_ _ _ _ _ _ _ w3962]
                  tunnel: w3726 -> [_ w3820 _ _ _ _ _ _]
                  tunnel: w3725 -> [_ _ w3847 _ _ _ _ _]
                  tunnel: w3724 -> [_ _ _ w3875 _ _ _ _]
                  tunnel: w3723 -> [_ _ _ _ w3903 _ _ _]
                  tunnel: w3722 -> [_ _ _ _ _ w3931 _ _]
                  tunnel: w3721 -> [_ _ _ _ _ _ w3959 _]
                  tunnel: w3719 -> [_ _ w3846 w3874 w3902 w3930 w3958 w3964]
                  tunnel: T15 {"1  (A) cal"=1.0, "1 (V) cal"=1.0, "1 (PF) cal"=1.0, "1 (TL) cal"=1.0, "1 (TN) cal"=1.0, "2 (A) cal"=1.0, "2 (V) cal"=1.0, "2 (PF) cal"=1.0, "2 (TL) cal"=1.0, "2 (TN) cal"=1.0} ("CAL LAB01") -> [_ _ w3845 w3873 w3901 w3929 w3957 _]
                  tunnel: w3716 -> [_ _ _ _ _ _ _ w3963]
                  tunnel: w3715 -> [w3772 _ _ _ _ _ _ _]
                  tunnel: w3713 -> [_ w3799 _ _ _ _ _ _]
                  frame #0 {
                    n2143 = Index Array(array=w3772, index=2) -> (element=w3767:bool)
                    n2144 = Index Array(array=w3772, index=1) -> (element=w3768:bool)
                    n2145 = Index Array(array=w3772, index=0) -> (element=w3769:bool)
                    n2146 = local write "Error USB #2"(w3767) -> ()
                    n2147 = local write "Error USB #0"(w3769) -> ()
                    n2148 = local write "Error USB #1"(w3768) -> ()
                    n2149 = stacked-sequence {
                      tunnel: w3769 -> [w3776 _ _ _]
                      tunnel: w3768 -> [_ w3781 _ _]
                      tunnel: 0 -> [w3775 w3780 w3785 _]
                      tunnel: w3767 -> [_ _ w3786 _]
                      frame #0 {
                        n2150 = case shown="True" w3776 {
                          tunnel: w3775 -> [w3777 _]
                          frame False {
                            n2151 = local write "Er USB#0"(w3777) -> ()
                          }
                          frame True {
                            n2152 = local read "Er USB#0"() -> (w3779:dbl)
                            n2153 = Increment(x=w3779) -> (x+1=→"Er USB#0":dbl)
                          }
                        }
                      }
                      frame #1 {
                        n2154 = case shown="True" w3781 {
                          tunnel: w3780 -> [w3782 _]
                          frame False {
                            n2155 = local write "Er USB#1"(w3782) -> ()
                          }
                          frame True {
                            n2156 = local read "Er USB#1"() -> (w3784:dbl)
                            n2157 = Increment(x=w3784) -> (x+1=→"Er USB#1":dbl)
                          }
                        }
                      }
                      frame #2 {
                        n2158 = case shown="True" w3786 {
                          tunnel: w3785 -> [w3787 _]
                          frame False {
                            n2159 = local write "Er USB#2"(w3787) -> ()
                          }
                          frame True {
                            n2160 = local read "Er USB#2"() -> (w3789:dbl)
                            n2161 = Increment(x=w3789) -> (x+1=→"Er USB#2":dbl)
                          }
                        }
                      }
                      frame #3 {
                        w3795 = 10
                        n2162 = local read "Er USB#2"() -> (w3796:dbl)
                        n2163 = local read "Er USB#0"() -> (w3798:dbl)
                        n2164 = local read "Er USB#1"() -> (w3797:dbl)
                        n2165 = Greater Or Equal?(x=w3798, y=w3795) -> (x >= y?=w3793:bool)
                        n2166 = Greater Or Equal?(x=w3797, y=w3795) -> (x >= y?=w3792:bool)
                        n2167 = Greater Or Equal?(x=w3796, y=w3795) -> (x >= y?=w3791:bool)
                        n2168 = Or(x=w3793, y=w3792) -> (x .or. y?=w3794:bool)
                        n2169 = Or(x=w3794, y=w3791) -> (x .or. y?=→"Analog error":bool)
                      }
                    }
                  }
                  frame #1 {
                    # "display graph data on ADM page"
                    n2170 = local write "AI loop time"(w3799) -> ()
                    n2171 = local write "AI"(TRUE) -> ()
                    n2172 = Index Array(array=w3820, index=6) -> (element=→"LAB04-1 (GRAPH)":dynamicdata)
                    n2173 = Index Array(array=w3820, index=7) -> (element=→"LAB04-2 (GRAPH)":dynamicdata)
                    n2174 = Index Array(array=w3820, index=9) -> (element=→"LAB05-2 (GRAPH)":dynamicdata)
                    n2175 = Index Array(array=w3820, index=8) -> (element=→"LAB05-1 (GRAPH)":dynamicdata)
                    n2176 = Index Array(array=w3820, index=5) -> (element=→"LAB03-2 (GRAPH)":dynamicdata)
                    n2177 = Index Array(array=w3820, index=0) -> (element=→"LAB01-1 (GRAPH)":dynamicdata)
                    n2178 = Index Array(array=w3820, index=1) -> (element=→"LAB01-2 (GRAPH)":dynamicdata)
                    n2179 = Index Array(array=w3820, index=2) -> (element=→"LAB02-1 (GRAPH)":dynamicdata)
                    n2180 = Index Array(array=w3820, index=3) -> (element=→"LAB02-2 (GRAPH)":dynamicdata)
                    n2181 = Index Array(array=w3820, index=4) -> (element=→"LAB03-1 (GRAPH)":dynamicdata)
                  }
                  frame #2 {
                    n2182 = case shown="False" w3846 {
                      tunnel: [w3848 w3849] -> w3844
                      tunnel: w3845 -> [_ w3849]
                      frame False {
                        n2183 = local read "CAL LAB01"() -> (w3848:T15)
                      }
                      frame True {
                      }
                    }
                    n2184 = Unbundle By Name(w3847) -> ("OFF amps"=w3843:dbl, "VOLTS"=w3842:dbl, "PF"=w3841:dbl, "OFF amps"=w3840:dbl, "VOLTS"=w3839:dbl, "PF"=w3838:dbl)
                    n2185 = Unbundle By Name(w3844) -> ("1  (A) cal"=w3837:dbl, "1 (V) cal"=w3836:dbl, "1 (PF) cal"=w3835:dbl, "2 (A) cal"=w3834:dbl, "2 (V) cal"=w3833:dbl, "2 (PF) cal"=w3832:dbl)  [unwired: 4 out]
                    n2186 = Multiply(x=w3843, y=w3837) -> (x*y=w3830:dbl)
                    n2187 = Multiply(x=w3842, y=w3836) -> (x*y=w3829:dbl)
                    n2188 = Multiply(x=w3841, y=w3835) -> (x*y=w3828:dbl)
                    n2189 = Multiply(x=w3840, y=w3834) -> (x*y=w3826:dbl)
                    n2190 = Multiply(x=w3839, y=w3833) -> (x*y=w3825:dbl)
                    n2191 = Multiply(x=w3838, y=w3832) -> (x*y=w3824:dbl)
                    n2192 = local read "SIG LAB01-2"() -> (w3827:T2)
                    n2193 = local read "SIG LAB01-1"() -> (w3831:T2)
                    n2194 = Bundle By Name(cluster=w3831, "AMPS"=w3830, "VOLTS"=w3829, "PF"=w3828) -> (w3823:T2)
                    n2195 = Bundle By Name(cluster=w3827, "AMPS"=w3826, "VOLTS"=w3825, "PF"=w3824) -> (w3822:T2)
                    n2196 = global write "Global display 1.vi" "SIG LAB01-2"(w3822) -> ()
                    n2197 = global write "Global display 1.vi" "SIG LAB01-1"(w3823) -> ()
                    n2198 = local write "SIG LAB01-2"(w3822) -> ()
                    n2199 = local write "SIG LAB01-1"(w3823) -> ()
                  }
                  frame #3 {
                    n2200 = Unbundle By Name(w3875) -> ("OFF amps"=w3871:dbl, "VOLTS"=w3870:dbl, "PF"=w3869:dbl, "OFF amps"=w3868:dbl, "VOLTS"=w3867:dbl, "PF"=w3866:dbl)
                    n2201 = case shown="True" w3874 {
                      tunnel: [w3876 w3877] -> w3872
                      tunnel: w3873 -> [_ w3877]
                      frame False {
                        n2202 = local read "CAL LAB02"() -> (w3876:T16)
                      }
                      frame True {
                      }
                    }
                    n2203 = Unbundle By Name(w3872) -> ("1  (A) cal"=w3865:dbl, "1 (V) cal"=w3864:dbl, "1 (PF) cal"=w3863:dbl, "2 (A) cal"=w3862:dbl, "2 (V) cal"=w3861:dbl, "2 (PF) cal"=w3860:dbl)  [unwired: 4 out]
                    n2204 = Multiply(x=w3871, y=w3865) -> (x*y=w3858:dbl)
                    n2205 = Multiply(x=w3870, y=w3864) -> (x*y=w3857:dbl)
